vi "Format Text From Progress State.vi"(5 "Procedure type":T2, 6 "Glue Procedure Steps":T1, 7 "Start/End":enum16{"Start", "End"}(ring)=enum."End", 10 "Canceled":bool, 11 "Potting Progress States":T3) -> (3 "String":string)   [LabVIEW 2011]
uses:
  Potting Application/UI typedefs/Progress States.ctl
  Shared Components/WorkTable Class/Type Definitions/Worktable_Mode.ctl
  Gluing Application/UI typedefs/Glue Progress States.ctl
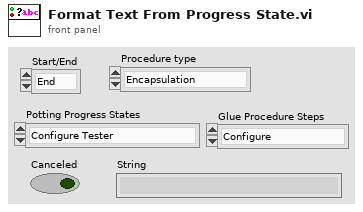
[diagram p1: front panel]
types:
  T1 = typedef "Glue Progress States.ctl" = enum16{"Configure", "Inspect Fuducials", "Review Fuducials", "Prepare Glue", "Stamping", "HDI Placement", "Weight Placement", "Finish"}
  T2 = typedef "Worktable_Mode.ctl" = enum16{"Encapsulation", "Gluing"}
  T3 = typedef "Progress States.ctl" = enum16{"Configure Tester", "Inspect Fiducials", "Review Fiducials", "Inspect Modules", "Review Modules", "Fill Sylgard", "Align Needle", "Purge", "Pot", "Finish"}
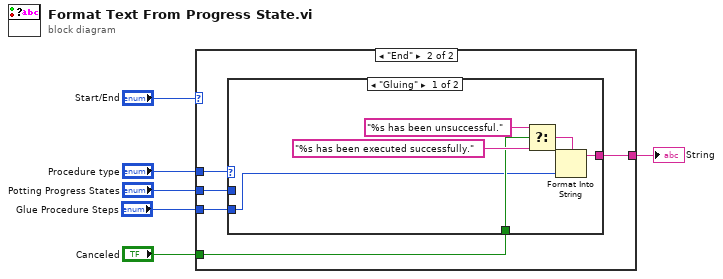
[diagram p0: block diagram]
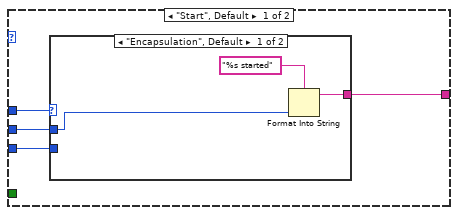
[diagram p2: hidden frame]
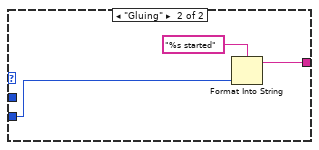
[diagram p3: hidden frame]
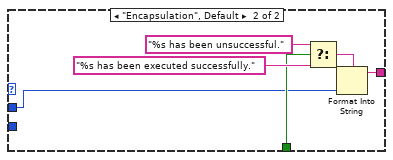
[diagram p4: hidden frame]
diagram:
  n1 = case shown="\"End\"" "Start/End" {
    tunnel: "Canceled" -> [_ w21]
    tunnel: [w9 w20] -> w5
    tunnel: "Procedure type" -> [w10 w19]
    tunnel: "Potting Progress States" -> [w8 w18]
    tunnel: "Glue Procedure Steps" -> [w7 w17]
    frame "Start", Default {
      n2 = case shown="\"Encapsulation\", Default" w10 {
        tunnel: [w12 w15] -> w9
        tunnel: w8 -> [w11 _]
        tunnel: w7 -> [_ w14]
        frame "Encapsulation", Default {
          n3 = Format Into String(format string="%s started" ("t"), w11) -> (resulting string=w12:string)  [unwired: 2 in, 1 out]
        }
        frame "Gluing" {
          n4 = Format Into String(format string="%s started" ("t"), w14) -> (resulting string=w15:string)  [unwired: 2 in, 1 out]
        }
      }
    }
    frame "End" {
      n5 = case shown="\"Gluing\"" w19 {
        tunnel: w21 -> [w24 w30]
        tunnel: [w23 w29] -> w20
        tunnel: w18 -> [_ w28]
        tunnel: w17 -> [w22 _]
        frame "Gluing" {
          n6 = Select(t="%s has been unsuccessful.", s=w24, f="%s has been executed successfully." ("format string")) -> (s? t:f=w26:string)
          n7 = Format Into String(format string=w26, w22) -> (resulting string=w23:string)  [unwired: 2 in, 1 out]
        }
        frame "Encapsulation", Default {
          n8 = Select(t="%s has been unsuccessful.", s=w30, f="%s has been executed successfully." ("format string")) -> (s? t:f=w32:string)
          n9 = Format Into String(format string=w32, w28) -> (resulting string=w29:string)  [unwired: 2 in, 1 out]
        }
      }
    }
  }
  "String" <- w5
